vi "Set Base Pathvi.vi"(8 "error in (no error)":errorcluster, 11 "Base Path":path) -> (0 "error out":errorcluster)   [LabVIEW 2021, in "Path Utilities.lvlib"]
doc: "Setup the base path to append at each location (ProgramFiles, ProgramData, ...).\nUse the pallette VIs to obtain full paths individually.\neg: \"C:\\Public\\Document\\My\\Base\\Path\"\n\nSetting \"Show Available Paths\" to true will fill \"Available Paths\" array with all full paths available."
uses:
  Path Utilities.lvlib
  TypeDefs/FGV State.ctl
panel:
  out "Available Paths":path[](array[path])
  in  "Show Available Paths (F)":bool
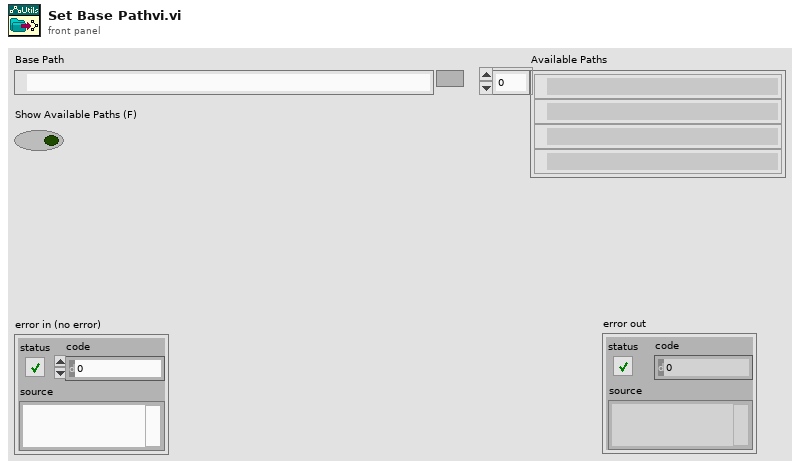
[diagram p1: front panel]
types:
  T1 = typedef "Path Utilities.lvlib/FGV State.ctl" = enum16{"Set Base Path", "Get Program Files", "Get Program Data", "Get App Data Local", "Get App Data Roaming", "Get User Documents", "Get Public Documents"}
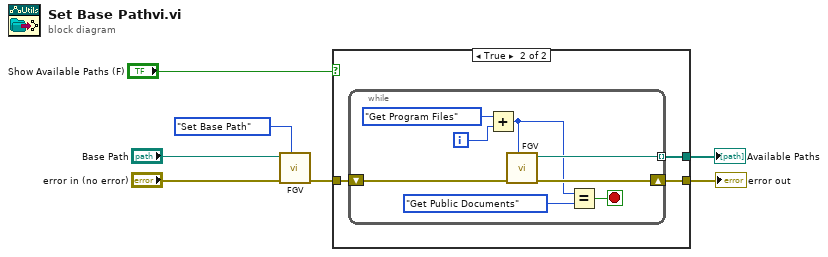
[diagram p0: block diagram]
diagram:
  n1 = call "FGV.vi"("FGV State"=FGV_State."Set Base Path", "error in (no error)"="error in (no error)", "Path In"="Base Path") -> ("error out"=w4:errorcluster)  [unwired: 7 in, 1 out]
  n2 = case shown="True" "Show Available Paths (F)" {
    tunnel: w4 -> [w8 w11]
    tunnel: [w8 w10] -> w2
    tunnel: [_ w9] -> w1
    frame False {
    }
    frame True {
      n3 = while {
        shift-right: [w18] -> w10
        shift-left: w11 -> [w19]
        tunnel: [w17] -> w9 mode=indexing
        i -> [w15]
        stop <- w12 stop-if-true
        n4 = Add(x=FGV_State."Get Program Files" ("FGV State"), y=w15) -> (x+y=w13:i32)
        n5 = call "FGV.vi"("FGV State"=w13, "error in (no error)"=w19) -> ("error out"=w18:errorcluster, "Path Out"=w17:path)  [unwired: 8 in]
        n6 = Equal?(x=w13, y=FGV_State."Get Public Documents" ("FGV State")) -> (x = y?=w12:bool)
      }
    }
  }
  "error out" <- w2
  "Available Paths" <- w1
